vi "events.get.vi"(11 "client in":refnum<class "client.lvclass">) -> (2 "events":T1, 3 "client out":refnum<class "client.lvclass">)   [LabVIEW 2020, in "client.lvclass"]
uses:
  client.lvclass
  client.lvclass/client.ctl
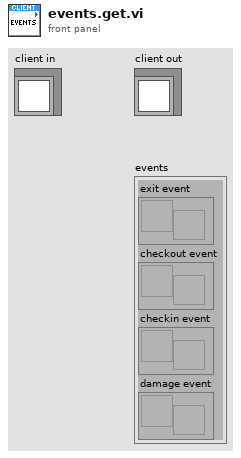
[diagram p1: front panel]
types:
  T1 = cluster{"exit event":refnum<user-event>, "checkout event":refnum<user-event>, "checkin event":refnum<user-event>, "damage event":refnum<user-event>}
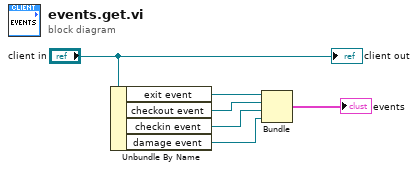
[diagram p0: block diagram]
diagram:
  n1 = Unbundle By Name("client in") -> ("exit event"=w5:refnum<user-event>, "checkout event"=w4:refnum<user-event>, "checkin event"=w3:refnum<user-event>, "damage event"=w2:refnum<user-event>)
  n2 = Bundle("exit event"=w5, "checkout event"=w4, "checkin event"=w3, "damage event"=w2) -> (→"events":T1)  [unwired: 1 in]
  "client out" <- "client in"
